vi "add list channel to configuration.vi"(6 "channel classification":T1, 7 "element name":string, 8 "error in (no error)":errorcluster, 9 "data type":T2, 10 "node ref":refnum<data-value>, 11 "engine ref":refnum<data-value>) -> (0 "error out":errorcluster)   [LabVIEW 2013, in "Shared Memory editor node.lvclass"]
uses:
  Shared Memory editor node.lvclass
  <vilib>/NI/DCAF/Tag Editor Core/Configuration Editor/Classes/Module editor node/module editor node.lvclass
  <vilib>/NI/Tag Bus/tag/Data Type.ctl
  <vilib>/NI/Tag Bus Module Framework/channel/channel classification.ctl
  <vilib>/NI/DCAF/Tag Editor Core/Configuration Editor/Classes/Engine Parent/Engine Parent Editor Node.lvclass
  <vilib>/NI/Configuration Framework/serializable configuration/NISE_CEF_serializable configuration.lvclass/NISE_CEF_serializable configuration.ctl
  <vilib>/Utility/LVClass/Get LV Class Name.vi
  <vilib>/NI/Configuration Framework/error generator/NISE_error generator.vi
  <vilib>/NI/Tag Bus Module Framework/channel/TBM channel.lvclass
  <vilib>/NI/Module Execution Interface/Engine Configuration/engine configuration.lvclass
  <vilib>/NI/Configuration Framework/serializable configuration/NISE_CEF_serializable configuration.lvclass
  module/configuration/Shared Memory configuration.lvclass
  <vilib>/NI/Tag Bus/tag/tag descriptor.lvclass
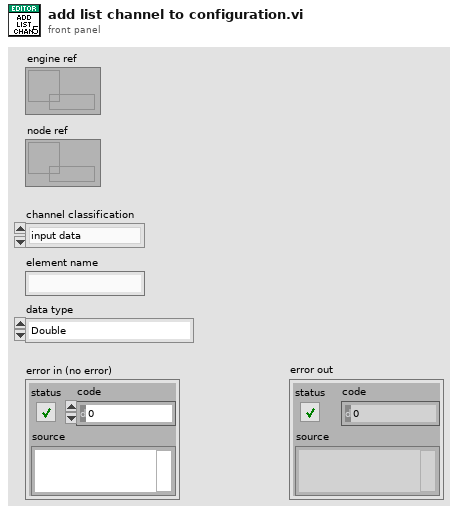
[diagram p1: front panel]
types:
  T1 = typedef "TBM channel.lvclass/channel classification.ctl" = enum16{"input data", "output data", "processing parameter", "processing result"}
  T2 = typedef "tag bus.lvlib/tag descriptor.lvclass/Data Type.ctl" = enum16{"Double", "Single", "I64", "I32", "I16", "I8", "U64", "U32", "U16", "U8", "Boolean", "String", "Array of Double", "Array of Single", "Array of I64", "Array of I32", "Array of I16", "Array of I8", "Array of U64", "Array of U32", "Array of U16", "Array of U8", "Array of Boolean", "Array of String"}
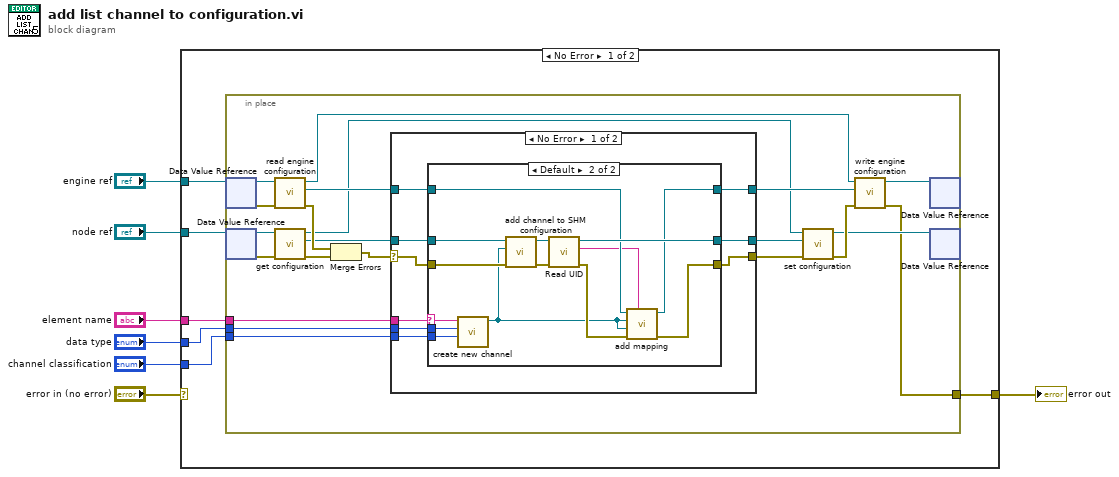
[diagram p0: block diagram]
diagram:
  n1 = case shown="No Error" "error in (no error)" {
    selector: "error in (no error)" -> [_ w64]
    tunnel: "node ref" -> [w13 _]
    tunnel: "engine ref" -> [w12 _]
    tunnel: "element name" -> [w11 _]
    tunnel: "channel classification" -> [w10 _]
    tunnel: "data type" -> [w9 _]
    tunnel: [w8 w64] -> w1
    frame No Error {
      n2 = in-place {
        in-place-border: w11 -> [w23]
        in-place-border: w9 -> [w22]
        in-place-border: w10 -> [w21]
        in-place-border: [w15] -> w8
        # "Replace the C header file directory destination in the module configuration."
        n3 = in-place-dvr #1(w12) -> (w34:refnum<class "Engine Parent Editor Node.lvclass">, w29:errorcluster)
        n4 = in-place-dvr #2(w13) -> (w30:refnum<class "module editor node.lvclass">, w27:errorcluster)
        n5 = call <vilib>:"read engine configuration.vi"("error in"=w29, "Engine Parent Editor Node in"=w34) -> ("error out"=w28:errorcluster, "engine configuration"=w32:refnum<class "engine configuration.lvclass">, "Engine Parent Editor Node out"=w18:refnum<class "Engine Parent Editor Node.lvclass">)  [unwired: 7 in]
        n6 = call "get configuration.vi"("error in (no error)"=w27, "shared memory editor node in"=w30) -> ("error out"=w25:errorcluster, "shm configuration out"=w20:refnum<class "Shared Memory configuration.lvclass">, "shared memory editor node out"=w14:refnum<class "module editor node.lvclass">)  [unwired: 7 in]
        n7 = Merge Errors(w28, w25) -> (w26:errorcluster)
        n8 = case shown="No Error" w26 {
          selector: w26 -> [w41 w61]
          tunnel: [w43 w61] -> w24
          tunnel: [w38 w63] -> w31
          tunnel: w32 -> [w39 w63]
          tunnel: w20 -> [w42 w62]
          tunnel: [w40 w62] -> w19
          tunnel: w23 -> [w37 _]
          tunnel: w22 -> [w36 _]
          tunnel: w21 -> [w35 _]
          frame No Error {
            n9 = case shown="Default" w37 {
              selector: w37 -> [_ w55]
              tunnel: [w45 w60] -> w43
              tunnel: [w46 w58] -> w40
              tunnel: w42 -> [w46 w53]
              tunnel: w41 -> [w45 w54]
              tunnel: w39 -> [w44 w49]
              tunnel: [w44 w48] -> w38
              tunnel: w36 -> [_ w52]
              tunnel: w35 -> [_ w51]
              frame "" {
              }
              frame Default {
                n10 = call <vilib>:"create new channel.vi"("channel classification"=w51, "data type"=w52, "channel name"=w55) -> ("channel"=w50:refnum<class "TBM channel.lvclass">)  [unwired: 8 in]
                n11 = call "add channel to SHM configuration.vi"("error in"=w54, "channel"=w50, "SHM configuration in"=w53) -> ("error out"=w57:errorcluster, "SHM configuration out"=w56:refnum<class "Shared Memory configuration.lvclass">)  [unwired: 7 in]
                n12 = call <vilib>:"Read UID.vi"("error in"=w57, "configuration in"=w56) -> ("error out"=w59:errorcluster, "instance id"=w47:string, "configuration out"=w58:refnum<class "Shared Memory configuration.lvclass">)  [unwired: 7 in]
                n13 = call <vilib>:"add mapping.vi"("owner ID"=w47, "error in"=w59, "channel"=w50, "tag descriptor"=w50, "engine configuration"=w49) -> ("error out"=w60:errorcluster, "engine configuration out"=w48:refnum<class "engine configuration.lvclass">)  [unwired: 5 in]
              }
            }
          }
          frame Error {
          }
        }
        n14 = call "set configuration.vi"("error in (no error)"=w24, "shm configuration in"=w19, "shared memory editor node in"=w14) -> ("error out"=w17:errorcluster, "shared memory editor node out"=w16:refnum<class "module editor node.lvclass">)  [unwired: 7 in]
        n15 = call <vilib>:"write engine configuration.vi"("error in"=w17, "engine configuration"=w31, "Engine Parent Editor Node in"=w18) -> ("error out"=w15:errorcluster, "Engine Parent Editor Node out"=w33:refnum<class "Engine Parent Editor Node.lvclass">)  [unwired: 7 in]
        n16 = in-place-dvr #1(w33) -> ()  [unwired: 2 out]
        n17 = in-place-dvr #2(w16) -> ()  [unwired: 2 out]
      }
    }
    frame Error {
    }
  }
  "error out" <- w1
